vi "ReleaseSampleDataQueue.vi"(8 "error in (no error)":errorcluster, 11 "AnalysisPluginsBase in":refnum<class "AnalysisPluginsBase.lvclass">) -> (0 "error out":errorcluster, 3 "AnalysisPluginsBase out":refnum<class "AnalysisPluginsBase.lvclass">)   [LabVIEW 2018, in "AnalysisPlugins.lvlib" / "AnalysisPluginsBase.lvclass"]
uses:
  AnalysisPluginsBase.lvclass
  Typedefs/SampleDataInput.ctl
  Typedefs/clWindowData.ctl
  AnalysisPluginsBase.lvclass/AnalysisPluginsBase.ctl
  Accessors/Read SampleDataQueName.vi
  Accessors/Write SampleDataInput.vi
  Accessors/Write Window.vi
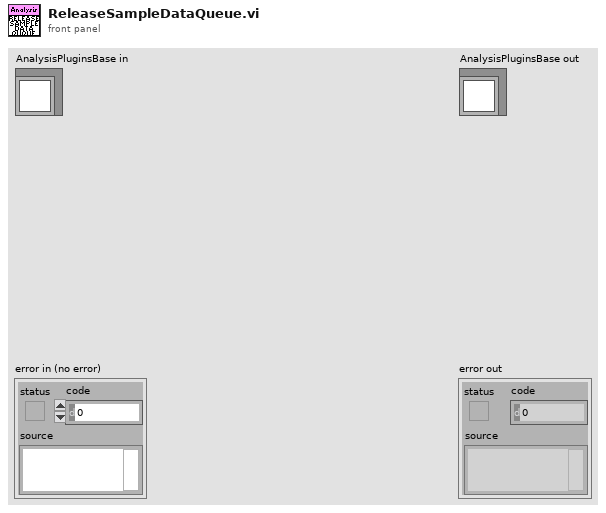
[diagram p1: front panel]
types:
  T1 = typedef "AnalysisPlugins.lvlib/AnalysisPluginsBase.lvclass/clWindowData.ctl" = cluster{"Timestamp":ext, "Samples":dbl[][], "Window Valid":bool, "T0":ext}
  T2 = typedef "AnalysisPlugins.lvlib/AnalysisPluginsBase.lvclass/SampleDataInput.ctl" = waveform(dbl)[]
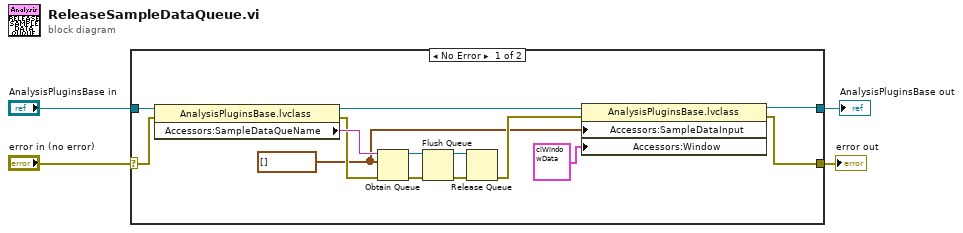
[diagram p0: block diagram]
diagram:
  n1 = case shown="No Error" "error in (no error)" {
    selector: "error in (no error)" -> [w6 w20]
    tunnel: [w5 w20] -> w3
    tunnel: [w7 w19] -> w1
    tunnel: "AnalysisPluginsBase in" -> [w8 w19]
    frame No Error {
      w10 = T2 [] ("clSampleDataArray")
      n2 = property class="AnalysisPluginsBase.lvclass"(reference=w8, error in=w6) -> (reference out=w12:refnum<class "AnalysisPluginsBase.lvclass">, error out=w17:errorcluster, "Accessors:SampleDataQueName"=w18:string)
      n3 = Obtain Queue(name (unnamed)=w18, element data type=w10, error in (no error)=w17) -> (queue out=w15:refnum<queue>, error out=w16:errorcluster)  [unwired: 2 in, 1 out]
      n4 = Flush Queue(queue=w15, error in (no error)=w16) -> (queue out=w13:refnum<queue>, error out=w14:errorcluster)  [unwired: 1 out]
      n5 = Release Queue(queue=w13, error in (no error)=w14) -> (error out=w11:errorcluster)  [unwired: 1 in, 2 out]
      n6 = property class="AnalysisPluginsBase.lvclass"(reference=w12, error in=w11, "Accessors:SampleDataInput"=w10, "Accessors:Window"=T1 {"Timestamp"=0.0, "Samples"=[], "Window Valid"=FALSE, "T0"=0.0} ("Window")) -> (reference out=w7:refnum<class "AnalysisPluginsBase.lvclass">, error out=w5:errorcluster)
    }
    frame Error {
    }
  }
  "error out" <- w3
  "AnalysisPluginsBase out" <- w1
